vi "Limelight Seeking Target.vi"() -> (0 "DriveCommand":dbl(knob)=-0.0 scale=-1.0..1.0, 1 "SteerCommand":dbl(knob)=nan scale=-1.0..1.0, 3 "TargetValid":bool)   [LabVIEW 2020]
uses:
  Robot Global Data.vi
panel:
  out "Drive Command Display":dbl format="%_6g"
  out "Steer Command Display":dbl format="%_6g"
  out "Steering Adjust":dbl
  out "Limelight tv":dbl
  out "Limelight ta":dbl
  out "Limelight tx":dbl
  out "MaxDrive":dbl(slide)=0.6824817518248175 min=0.0 max=1.0 step=0.01 scale=0.0..1.0
  out "DriveK":dbl(slide)=0.26277372262773724 min=0.0 max=1.0 step=0.05 scale=0.0..1.0
  out "Limelight Goal Area":dbl(slide)=14.872262773722628 min=0.1 max=25.0 step=0.25 scale=0.0..25.0
  out "AimDeadband":dbl min=0.0 max=10.0 step=0.25
  out "MinSteerCommand":dbl(slide)=0.2717391304347826 min=0.0 max=0.5 step=0.05 scale=0.0..0.5
  out "SteeringK":dbl(slide)=0.025362318840579712 min=0.0 max=0.25 step=0.01 scale=0.0..0.25
  # "// These numbers must be tuned for your Robot!  Be careful!\n\n final double STEER_K = 0.03;                    \n// how hard to turn toward the target\n\n\n\n\n \n\nfinal double DESIRED_TARGET_AREA = 13.0;        \n// Area of the target when the robot reaches the wall\n\n\n\nfinal double DRIVE_K = 0.26;                   \n // how hard to drive fwd toward the target\n\n \n \nfinal double MAX_DRIVE = 0.7;                   \n// Simple speed limit so we don't drive too fast"
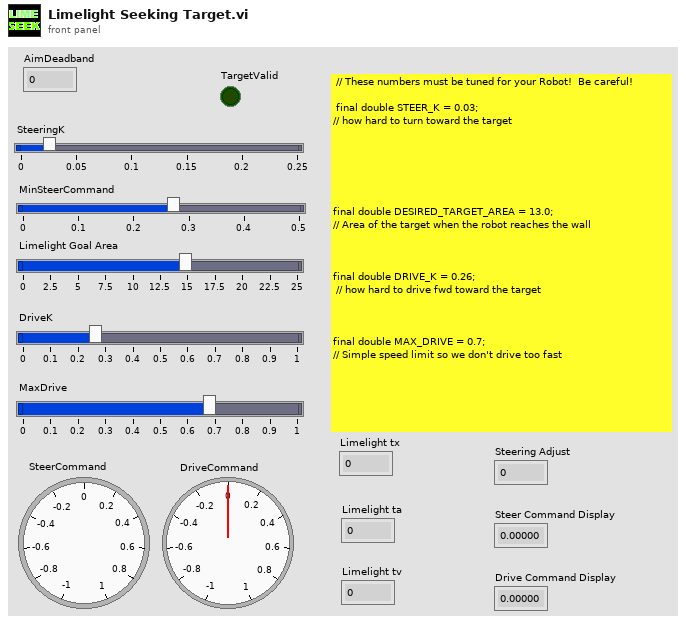
[diagram p1: front panel]
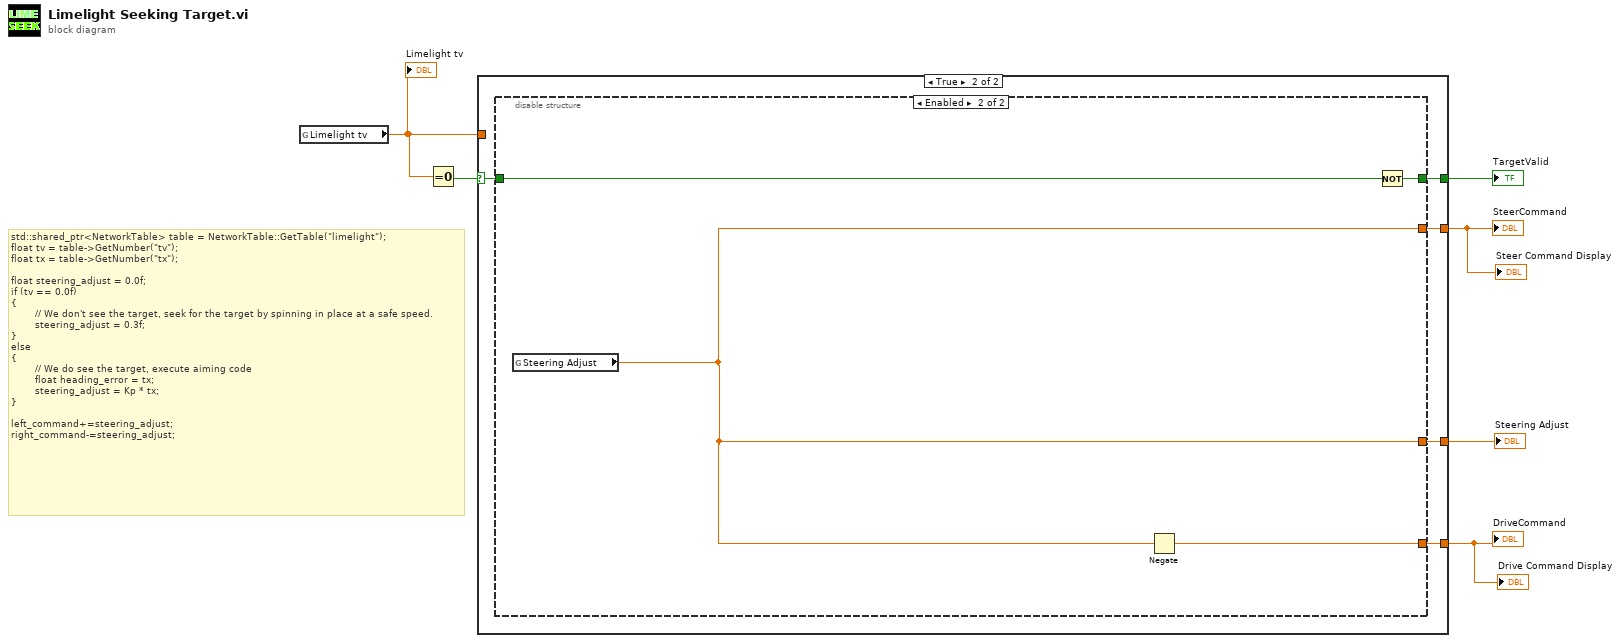
[diagram p0: block diagram]
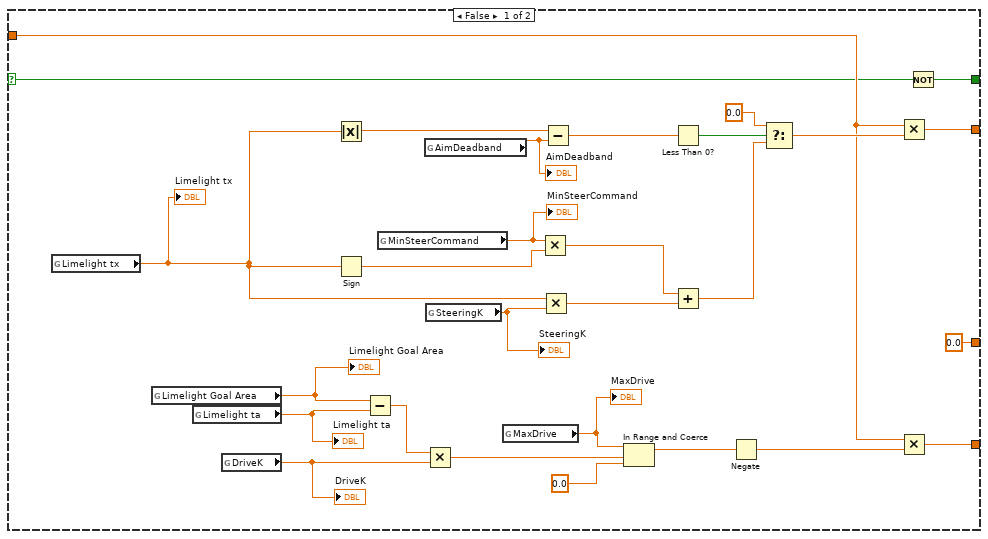
[diagram p2: hidden frame]
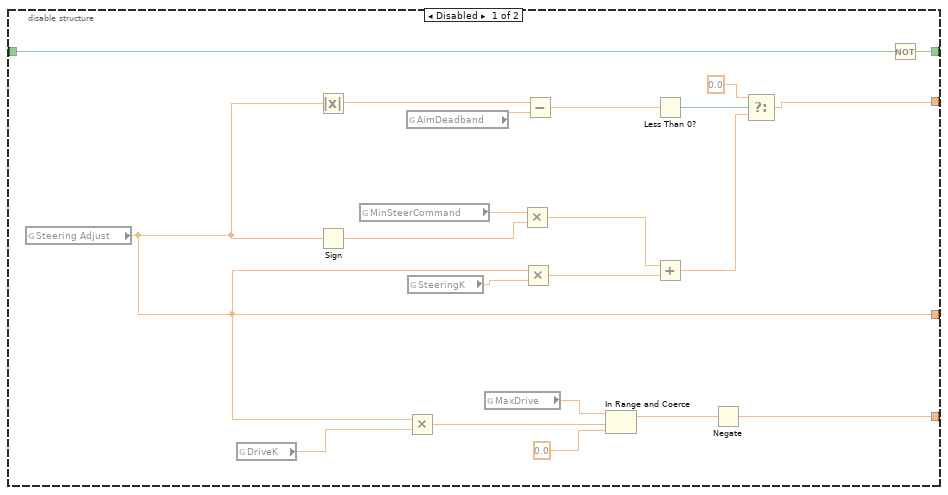
[diagram p3: hidden frame]
diagram:
  # "std::shared_ptr<NetworkTable> table = NetworkTable::GetTable(\"limelight\");\nfloat tv = table->GetNumber(\"tv\");\nfloat tx = table->GetNumber(\"tx\");\n\nfloat steering_adjust = 0.0f;\nif (tv == 0.0f)\n{\n        // We don't see the target, seek for the target by spinning in place at a safe speed.\n        steering_adjust = 0.3f;\n}\nelse\n{\n        // We do see the target, execute aiming code\n        float heading_error = tx;\n        steering_adjust = Kp * tx;\n}\n\nleft_command+=steering_adjust;\nright_command-=steering_adjust;"
  n1 = global read "Robot Global Data.vi" "Limelight tv"() -> (w4:dbl)
  "Limelight tv" <- w4
  n2 = Equal To 0?(x=w4) -> (x = 0?=w6:bool)
  n3 = case shown="True" w6 {
    selector: w6 -> [w9 w37]
    tunnel: [w27 w39] -> w3
    tunnel: [w22 w38] -> w2
    tunnel: w4 -> [w11 _]
    tunnel: [w8 w36] -> w5
    tunnel: [0.0 ("Steering Adjust") w35] -> w1
    frame False {
      n4 = global read "Robot Global Data.vi" "Limelight tx"() -> (w18:dbl)
      "Limelight tx" <- w18
      n5 = global read "Robot Global Data.vi" "Limelight Goal Area"() -> (w10:dbl)
      "Limelight Goal Area" <- w10
      n6 = global read "Robot Global Data.vi" "Limelight ta"() -> (w17:dbl)
      "Limelight ta" <- w17
      n7 = global read "Robot Global Data.vi" "DriveK"() -> (w16:dbl)
      "DriveK" <- w16
      n8 = Absolute Value(x=w18) -> (abs(x)=w31:dbl)
      n9 = Sign(1:w18) -> (0:w26:dbl)
      n10 = Subtract(x=w10, y=w17) -> (x-y=w25:dbl)
      n11 = global read "Robot Global Data.vi" "MinSteerCommand"() -> (w12:dbl)
      "MinSteerCommand" <- w12
      n12 = global read "Robot Global Data.vi" "AimDeadband"() -> (w13:dbl)
      "AimDeadband" <- w13
      n13 = Multiply(x=w25, y=w16) -> (x*y=w24:dbl)
      n14 = global read "Robot Global Data.vi" "SteeringK"() -> (w15:dbl)
      "SteeringK" <- w15
      n15 = global read "Robot Global Data.vi" "MaxDrive"() -> (w14:dbl)
      "MaxDrive" <- w14
      n16 = Multiply(x=w12, y=w26) -> (x*y=w30:dbl)
      n17 = Multiply(x=w18, y=w15) -> (x*y=w29:dbl)
      n18 = Subtract(x=w31, y=w13) -> (x-y=w32:dbl)
      n19 = In Range and Coerce(upper limit=w14, x=w24, lower limit=0.0) -> (coerced(x)=w21:dbl)  [unwired: 1 out]
      n20 = Less Than 0?(x=w32) -> (x < 0?=w33:bool)
      n21 = Add(x=w30, y=w29) -> (x+y=w19:dbl)
      n22 = Negate(x=w21) -> (-x=w20:dbl)
      n23 = Select(t=0.0, s=w33, f=w19) -> (s? t:f=w28:dbl)
      n24 = Multiply(x=w11, y=w28) -> (x*y=w27:dbl)
      n25 = Multiply(x=w11, y=w20) -> (x*y=w22:dbl)
      n26 = Not(x=w9) -> (.not. x?=w8:bool)
    }
    frame True {
      n27 = disable-structure shown="Enabled" {
        disable-tunnel: [w54 w62] -> w39
        disable-tunnel: [w49 w61] -> w38
        disable-tunnel: w37 -> [w42 w64]
        disable-tunnel: [w41 w63] -> w36
        disable-tunnel: [w40 w62] -> w35
        frame Disabled {
          n28 = global read "Robot Global Data.vi" "Steering Adjust"() -> (w40:dbl)
          n29 = global read "Robot Global Data.vi" "DriveK"() -> (w47:dbl)
          n30 = Absolute Value(x=w40) -> (abs(x)=w57:dbl)
          n31 = Sign(1:w40) -> (0:w53:dbl)
          n32 = global read "Robot Global Data.vi" "MinSteerCommand"() -> (w43:dbl)
          n33 = global read "Robot Global Data.vi" "AimDeadband"() -> (w44:dbl)
          n34 = Multiply(x=w40, y=w47) -> (x*y=w52:dbl)
          n35 = global read "Robot Global Data.vi" "SteeringK"() -> (w46:dbl)
          n36 = global read "Robot Global Data.vi" "MaxDrive"() -> (w45:dbl)
          n37 = Multiply(x=w43, y=w53) -> (x*y=w56:dbl)
          n38 = Multiply(x=w40, y=w46) -> (x*y=w55:dbl)
          n39 = Subtract(x=w57, y=w44) -> (x-y=w58:dbl)
          n40 = In Range and Coerce(upper limit=w45, x=w52, lower limit=0.0) -> (coerced(x)=w50:dbl)  [unwired: 1 out]
          n41 = Less Than 0?(x=w58) -> (x < 0?=w59:bool)
          n42 = Add(x=w56, y=w55) -> (x+y=w48:dbl)
          n43 = Negate(x=w50) -> (-x=w49:dbl)
          n44 = Select(t=0.0, s=w59, f=w48) -> (s? t:f=w54:dbl)
          n45 = Not(x=w42) -> (.not. x?=w41:bool)
        }
        frame Enabled {
          n46 = global read "Robot Global Data.vi" "Steering Adjust"() -> (w62:dbl)
          n47 = Negate(x=w62) -> (-x=w61:dbl)
          n48 = Not(x=w64) -> (.not. x?=w63:bool)
        }
      }
    }
  }
  "SteerCommand" <- w3
  "DriveCommand" <- w2
  "TargetValid" <- w5
  "Drive Command Display" <- w2
  "Steer Command Display" <- w3
  "Steering Adjust" <- w1
